vi "PathPlanner_PathFinder_ComputeOrImprovePath.vi"(8 "error in (no error)":errorcluster) -> (0 "error out":errorcluster)   [LabVIEW 2019, in "PathPlanner24.lvlib"]
uses:
  PathPlanner24.lvlib
  PathPlanner_GridPosition_FromHash.vi
  PathPlanner_PathFinder_Heuristic.vi
  PathPlanner_GridPosition_Get.vi
  PathPlanner_GridPosition_New.vi
  PathPlanner_PathFinder_Globals.vi
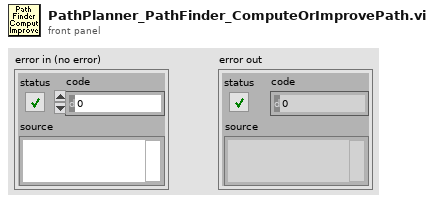
[diagram p1: front panel]
types:
  T1 = typedef "PathPlanner24.lvlib/PathPlannerFinderDoublePair.ctl" = cluster{"A":dbl, "B":dbl}
  T2 = typedef "PathPlanner24.lvlib/PathPlannerFinderGridPosition.ctl" = cluster{"X":i32, "Y":i32}
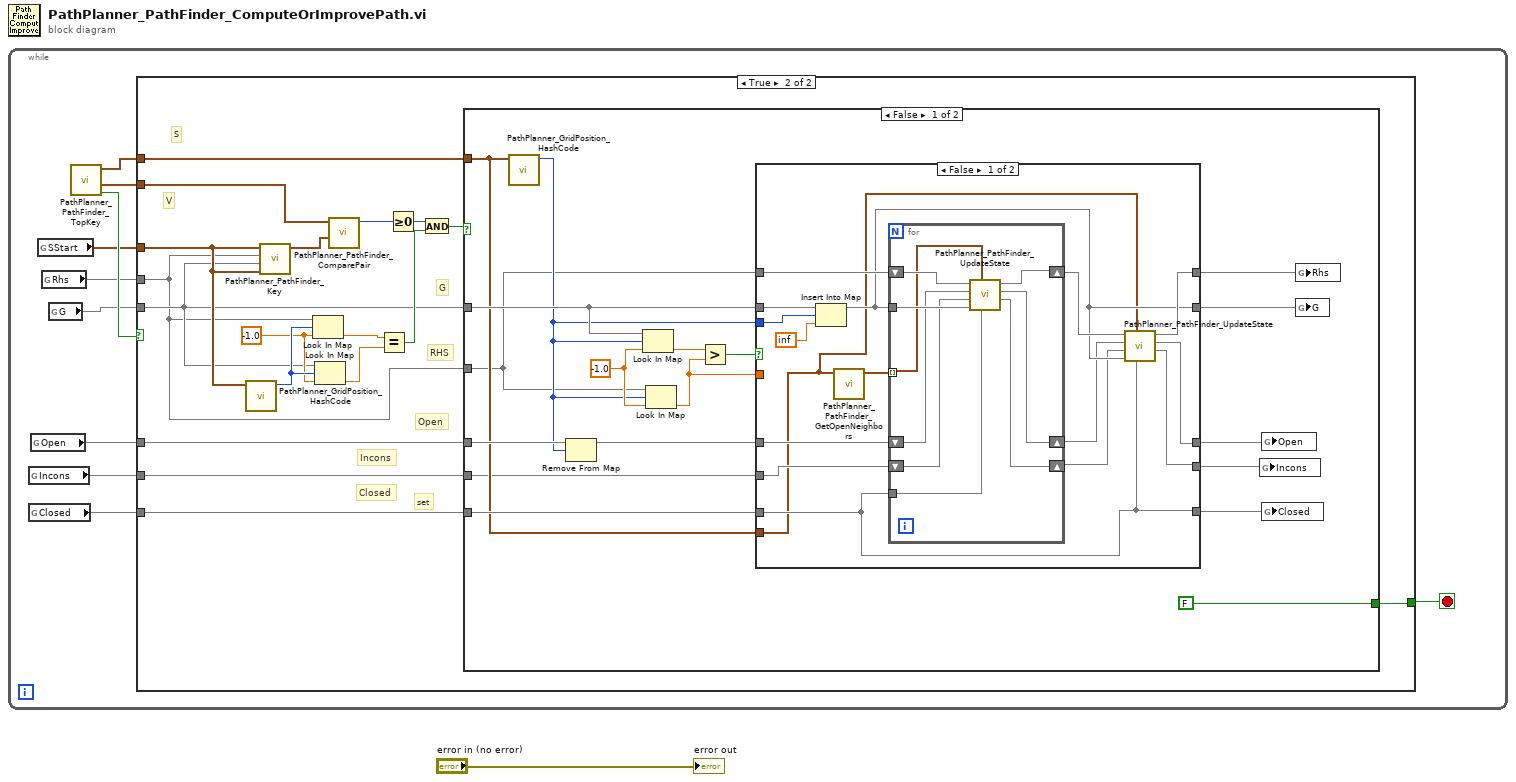
[diagram p0: block diagram]
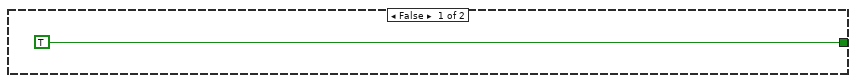
[diagram p2: hidden frame]
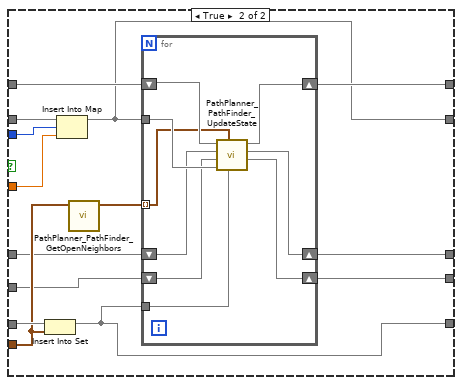
[diagram p3: hidden frame]
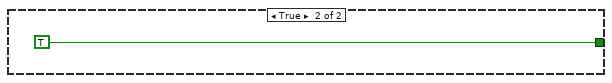
[diagram p4: hidden frame]
diagram:
  n1 = while {
    stop <- w10 stop-if-true
    n2 = global read "PathPlanner_PathFinder_Globals.vi" "Incons"() -> (w2:map{i32, T1})
    n3 = global read "PathPlanner_PathFinder_Globals.vi" "Closed"() -> (w3:set{T2})
    n4 = global read "PathPlanner_PathFinder_Globals.vi" "Open"() -> (w4:map{i32, T1})
    n5 = global read "PathPlanner_PathFinder_Globals.vi" "SStart"() -> (w7:T2)
    n6 = global read "PathPlanner_PathFinder_Globals.vi" "Rhs"() -> (w6:map{i32, dbl})
    n7 = global read "PathPlanner_PathFinder_Globals.vi" "G"() -> (w5:map{i32, dbl})
    n8 = call "PathPlanner_PathFinder_TopKey.vi"() -> ("Found"=w11:bool, "DoublePair"=w8:T1, "PathPlannerFinderGridPosition"=w9:T2)  [unwired: 9 in]
    n9 = case shown="True" w11 {
      tunnel: [TRUE w19] -> w10
      tunnel: w9 -> [_ w17]
      tunnel: w8 -> [_ w30]
      tunnel: w7 -> [_ w26]
      tunnel: w6 -> [_ w15]
      tunnel: w5 -> [_ w16]
      tunnel: w4 -> [_ w18]
      tunnel: w3 -> [_ w14]
      tunnel: w2 -> [_ w13]
      frame False {
      }
      frame True {
        w24 = -1.0 ("default value")
        # "Incons"
        # "set"
        # "Closed"
        # "RHS"
        # "Open"
        # "G"
        # "S"
        # "V"
        n10 = call "PathPlanner_GridPosition_HashCode.vi"("GridPosition"=w26) -> ("HashCode"=w25:i32)  [unwired: 10 in]
        n11 = call "PathPlanner_PathFinder_Key.vi"("Sstart"=w26, "G"=w16, "RHS"=w15, "S"=w26) -> ("DoublePair"=w29:T1)  [unwired: 7 in]
        n12 = Look In Map(map=w15, key=w25, default value=w24) -> (value=w23:dbl)  [unwired: 1 out]
        n13 = Look In Map(map=w16, key=w25, default value=w24) -> (value=w22:dbl)  [unwired: 1 out]
        n14 = call "PathPlanner_PathFinder_ComparePair.vi"("B"=w29, "A"=w30) -> ("Compare"=w28:i32)  [unwired: 9 in]
        n15 = Equal?(x=w23, y=w22) -> (x = y?=w21:bool)
        n16 = Greater Or Equal To 0?(x=w28) -> (x >= 0?=w27:bool)
        n17 = And(x=w27, y=w21) -> (x .and. y?=w20:bool)
        n18 = case shown="False" w20 {
          tunnel: [FALSE TRUE] -> w19
          tunnel: w18 -> [w48 _]
          tunnel: w17 -> [w40 _]
          tunnel: w16 -> [w44 _]
          tunnel: w15 -> [w39 _]
          tunnel: w14 -> [w41 _]
          tunnel: w13 -> [w37 _]
          frame False {
            w47 = -1.0 ("default value")
            n19 = call "PathPlanner_GridPosition_HashCode.vi"("GridPosition"=w40) -> ("HashCode"=w43:i32)  [unwired: 10 in]
            n20 = Remove From Map(10:w43, 11:w48) -> (3:w38:map{i32, T1})  [unwired: 2 out]
            n21 = Look In Map(map=w44, key=w43, default value=w47) -> (value=w46:dbl)  [unwired: 1 out]
            n22 = Look In Map(map=w39, key=w43, default value=w47) -> (value=w42:dbl)  [unwired: 1 out]
            n23 = Greater?(x=w46, y=w42) -> (0:w45:bool)
            n24 = case shown="False" w45 {
              tunnel: w44 -> [w64 w87]
              tunnel: w43 -> [w63 w86]
              tunnel: w42 -> [_ w85]
              tunnel: w41 -> [w50 w84]
              tunnel: w40 -> [w49 w83]
              tunnel: [w50 w75] -> w36
              tunnel: [w55 w74] -> w32
              tunnel: w39 -> [w61 w81]
              tunnel: [w56 w80] -> w33
              tunnel: w38 -> [w59 w79]
              tunnel: [w53 w78] -> w34
              tunnel: w37 -> [w58 w77]
              tunnel: [w51 w76] -> w35
              frame False {
                n25 = Insert Into Map(map in=w64, key=w63, value=inf) -> (map out=w55:map{i32, dbl})  [unwired: 2 out]
                n26 = call "PathPlanner_PathFinder_GetOpenNeighbors.vi"("GridPosition S"=w49) -> ("Neighbors"=w60:T2[])  [unwired: 10 in]
                n27 = for {
                  shift-right: [w72] -> w57
                  shift-left: w61 -> [w73]
                  shift-right: [w69] -> w54
                  shift-left: w59 -> [w70]
                  shift-right: [w67] -> w52
                  shift-left: w58 -> [w68]
                  tunnel: w60 -> [w65] mode=indexing
                  tunnel: w55 -> [w71]
                  tunnel: w50 -> [w66]
                  n28 = call "PathPlanner_PathFinder_UpdateState.vi"("Closed"=w66, "S"=w65, "G"=w71, "Incons"=w68, "Open"=w70, "RHS"=w73) -> ("Incons out"=w67:map{i32, T1}, "Open out"=w69:map{i32, T1}, "RHS out"=w72:map{i32, dbl})  [unwired: 3 in]
                }
                n29 = call "PathPlanner_PathFinder_UpdateState.vi"("Closed"=w50, "S"=w49, "G"=w55, "Incons"=w52, "Open"=w54, "RHS"=w57) -> ("Incons out"=w51:map{i32, T1}, "Open out"=w53:map{i32, T1}, "RHS out"=w56:map{i32, dbl})  [unwired: 3 in]
              }
              frame True {
                n30 = Insert Into Set(10:w83, 11:w84) -> (3:w75:set{T2})  [unwired: 1 out]
                n31 = Insert Into Map(map in=w87, key=w86, value=w85) -> (map out=w74:map{i32, dbl})  [unwired: 2 out]
                n32 = call "PathPlanner_PathFinder_GetOpenNeighbors.vi"("GridPosition S"=w83) -> ("Neighbors"=w82:T2[])  [unwired: 10 in]
                n33 = for {
                  tunnel: w82 -> [w89] mode=indexing
                  shift-right: [w95] -> w80
                  shift-left: w81 -> [w96]
                  shift-right: [w92] -> w78
                  shift-left: w79 -> [w93]
                  shift-right: [w90] -> w76
                  shift-left: w77 -> [w91]
                  tunnel: w74 -> [w94]
                  tunnel: w75 -> [w88]
                  n34 = call "PathPlanner_PathFinder_UpdateState.vi"("Closed"=w88, "S"=w89, "G"=w94, "Incons"=w91, "Open"=w93, "RHS"=w96) -> ("Incons out"=w90:map{i32, T1}, "Open out"=w92:map{i32, T1}, "RHS out"=w95:map{i32, dbl})  [unwired: 3 in]
                }
              }
            }
            n35 = global write "PathPlanner_PathFinder_Globals.vi" "Incons"(w35) -> ()
            n36 = global write "PathPlanner_PathFinder_Globals.vi" "Open"(w34) -> ()
            n37 = global write "PathPlanner_PathFinder_Globals.vi" "Closed"(w36) -> ()
            n38 = global write "PathPlanner_PathFinder_Globals.vi" "Rhs"(w33) -> ()
            n39 = global write "PathPlanner_PathFinder_Globals.vi" "G"(w32) -> ()
          }
          frame True {
          }
        }
      }
    }
  }
  "error out" <- "error in (no error)"
